vi "Schedule Polling.vi"(8 "error in (no error)":errorcluster, 11 "Instruments in":refnum<class "Instruments.lvclass">) -> (0 "error out":errorcluster, 3 "Instruments out":refnum<class "Instruments.lvclass">)   [LabVIEW 2023, in "Instruments.lvlib" / "Instruments.lvclass"]
doc: "Schedule periodic poll message at the defined poll rate\nThis is called in the post-actor routine."
uses:
  Library/Instruments.lvclass
  C:/Users/Public/Documents/Development/builds/Framework/Engine.lvlibp/Engine/Library/Engine.lvclass
  Instruments Messages/Measure Msg/Measure Msg.lvclass
  C:/Users/Public/Documents/Development/builds/Framework/Actor Framework.lvlibp/1abvi3w/vi.lib/ActorFramework/Message/Message.lvclass
  Library/Instruments.lvclass/Instruments.ctl
  builds/Framework/Engine.lvlibp/Engine/Accessors/Read Self Q.vi
  builds/Framework/Actor Framework.lvlibp/1abvi3w/vi.lib/ActorFramework/Message Enqueuer/Message Enqueuer.lvclass
  builds/Framework/Actor Framework.lvlibp
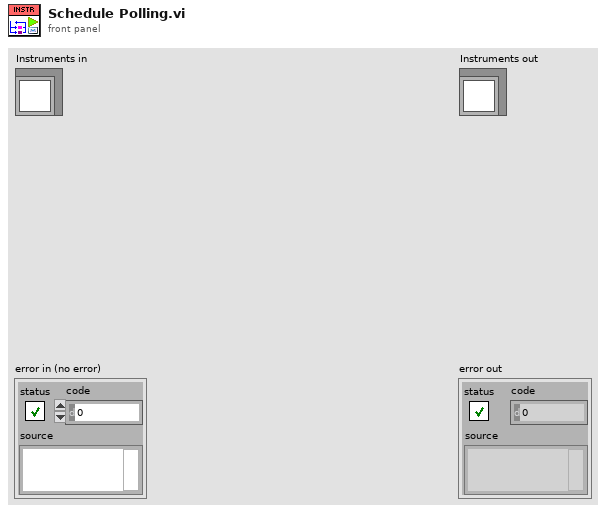
[diagram p1: front panel]
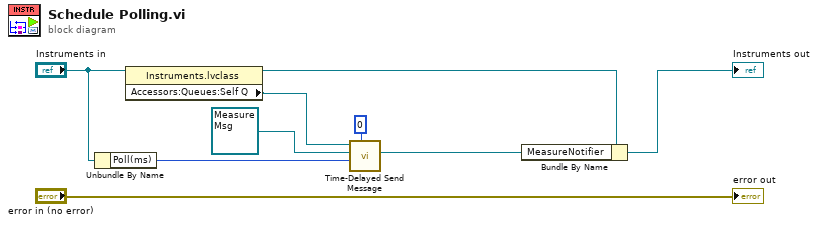
[diagram p0: block diagram]
diagram:
  n1 = Unbundle By Name("Instruments in") -> ("Poll(ms)"=w8:i32)
  n2 = property class="Instruments.lvclass"(reference="Instruments in") -> (reference out=w2:refnum<class "Instruments.lvclass">, "Accessors:Queues:Self Q"=w1:refnum<class "Message Enqueuer.lvclass">)  [unwired: 1 in, 1 out]
  n3 = call "Time-Delayed Send Message.vi"("# Copies (0 = infinite repeat)"=u32 0, "Milliseconds To Wait"=w8, "Message"=refnum<class "Measure Msg.lvclass"> refnum ("Instruments.lvlib:Measure Msg.lvclass"), "Message Enqueuer"=w1) -> ("Delivery Notifier"=w5:refnum<notifier>)  [unwired: 6 in, 1 out]
  n4 = Bundle By Name(cluster=w2, "MeasureNotifier"=w5) -> (→"Instruments out":refnum<class "Instruments.lvclass">)
  "error out" <- "error in (no error)"
